vi "ConfigDevice.vi"(8 "error in (no error)":errorcluster, 11 "ChromaPowerSupply in":refnum<class "ChromaPowerSupply.lvclass">) -> (0 "error out":errorcluster, 3 "ChromaPowerSupply out":refnum<class "ChromaPowerSupply.lvclass">)   [LabVIEW 2018, in "AcPwrPlugins.lvlib" / "ChromaPowerSupply.lvclass"]
doc: "This VI configures all the properties set by the user through the INI file or the Properties Dialog box."
uses:
  ChromaPowerSupply.lvclass
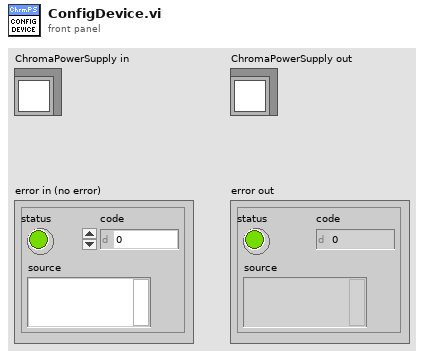
[diagram p1: front panel]
types:
  T1 = typedef "AcPwrPlugins.lvlib/ChromaPowerSupply.lvclass/Device(s)Settings.ctl" = cluster{"Phases":cluster{"Handle":string, "Instrument Options":string, "id query (T)":bool, "reset device (T)":bool, "Timing":cluster{"TimingOn":enum16{""}, "Hours":u32, "Minutes":u32, "Seconds":dbl, "CutoffVoltage":dbl}, "Connected":bool, "Output Mode":enum16{"Voltage (DC)", "Current (DC)"}, "Voltage":dbl, "Current":dbl, "High Voltage Limit":dbl, "High Current Limit":dbl, "Power Protect":dbl, "Current Protect":dbl, "Voltage Protect":dbl, "Low Current Limit":dbl, "Low Voltage Limit":dbl, "Current Slew Rate":dbl, "Voltage Slew Rate":dbl}[], "MeasName":string}
  T2 = cluster{"Handle":string, "Instrument Options":string, "id query (T)":bool, "reset device (T)":bool, "Timing":cluster{"TimingOn":enum16{""}, "Hours":u32, "Minutes":u32, "Seconds":dbl, "CutoffVoltage":dbl}, "Connected":bool, "Output Mode":enum16{"Voltage (DC)", "Current (DC)"}, "Voltage":dbl, "Current":dbl, "High Voltage Limit":dbl, "High Current Limit":dbl, "Power Protect":dbl, "Current Protect":dbl, "Voltage Protect":dbl, "Low Current Limit":dbl, "Low Voltage Limit":dbl, "Current Slew Rate":dbl, "Voltage Slew Rate":dbl}[]
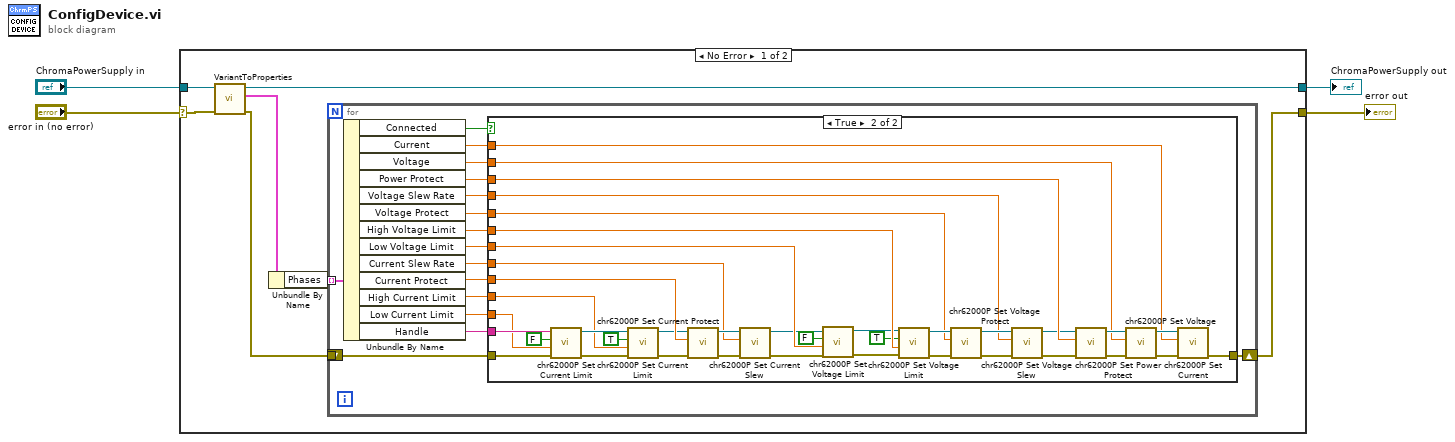
[diagram p0: block diagram]
diagram:
  n1 = case shown="No Error" "error in (no error)" {
    selector: "error in (no error)" -> [w10 w67]
    tunnel: "ChromaPowerSupply in" -> [w11 w68]
    tunnel: [w9 w68] -> w2
    tunnel: [w5 w67] -> w1
    frame No Error {
      n2 = call-dynamic "VariantToProperties.vi"("error in (no error)"=w10, "ChromaPowerSupply in"=w11) -> ("error out"=w6:errorcluster, "Device Settings"=w8:T1, "ChromaPowerSupply out"=w9:refnum<class "ChromaPowerSupply.lvclass">)  [unwired: 5 in, 2 out]
      n3 = Unbundle By Name(w8) -> ("Phases"=w7:T2)
      n4 = for {
        tunnel: w7 -> [w27] mode=indexing
        tunnel: w6 -> [w25]
        shift-right: [w22] -> w5
        shift-left: _ -> [_]
        n5 = Unbundle By Name(w27) -> ("Connected"=w18:bool, "Current"=w16:dbl, "Voltage"=w17:dbl, "Power Protect"=w19:dbl, "Voltage Slew Rate"=w12:dbl, "Voltage Protect"=w21:dbl, "High Voltage Limit"=w23:dbl, "Low Voltage Limit"=w14:dbl, "Current Slew Rate"=w13:dbl, "Current Protect"=w20:dbl, "High Current Limit"=w15:dbl, "Low Current Limit"=w24:dbl, "Handle"=w26:string)
        n6 = case shown="True" w18 {
          tunnel: w26 -> [_ w66]
          tunnel: w25 -> [w28 w65]
          tunnel: w24 -> [_ w61]
          tunnel: w23 -> [_ w64]
          tunnel: [w28 w51] -> w22
          tunnel: w21 -> [_ w57]
          tunnel: w20 -> [_ w60]
          tunnel: w19 -> [_ w56]
          tunnel: w17 -> [_ w50]
          tunnel: w16 -> [_ w49]
          tunnel: w15 -> [_ w43]
          tunnel: w14 -> [_ w40]
          tunnel: w13 -> [_ w36]
          tunnel: w12 -> [_ w29]
          frame False {
          }
          frame True {
            n7 = call <instrlib>:"chr62000P Set Current Limit.vi"("error in (no error)"=w65, "Current Limit (0.0)"=w61, "High/Low (Low)"=FALSE, "instrument handle"=w66) -> ("error out"=w48:errorcluster, "instrument handle out"=w47:refnum<k15>)  [unwired: 6 in]
            n8 = call <instrlib>:"chr62000P Set Current Limit.vi"("error in (no error)"=w48, "Current Limit (0.0)"=w43, "High/Low (Low)"=TRUE, "instrument handle"=w47) -> ("error out"=w45:errorcluster, "instrument handle out"=w46:refnum<k15>)  [unwired: 6 in]
            n9 = call <instrlib>:"chr62000P Set Current Protect.vi"("error in (no error)"=w45, "Current Protect (63.0)"=w60, "instrument handle"=w46) -> ("error out"=w38:errorcluster, "instrument handle out"=w37:refnum<k15>)  [unwired: 7 in]
            n10 = call <instrlib>:"chr62000P Set Current Slew.vi"("error in (no error)"=w38, "Current Slew (1.00)"=w36, "instrument handle"=w37) -> ("error out"=w34:errorcluster, "instrument handle out"=w35:refnum<k15>)  [unwired: 7 in]
            n11 = call <instrlib>:"chr62000P Set Voltage Limit.vi"("error in (no error)"=w34, "Voltage Limit (0.0)"=w40, "High/Low (Low)"=FALSE, "instrument handle"=w35) -> ("error out"=w41:errorcluster, "instrument handle out"=w42:refnum<k15>)  [unwired: 6 in]
            n12 = call <instrlib>:"chr62000P Set Voltage Limit.vi"("error in (no error)"=w41, "Voltage Limit (0.0)"=w64, "High/Low (Low)"=TRUE, "instrument handle"=w42) -> ("error out"=w59:errorcluster, "instrument handle out"=w58:refnum<k15>)  [unwired: 6 in]
            n13 = call <instrlib>:"chr62000P Set Voltage Protect.vi"("error in (no error)"=w59, "Voltage Protect (88.0)"=w57, "instrument handle"=w58) -> ("error out"=w33:errorcluster, "instrument handle out"=w32:refnum<k15>)  [unwired: 7 in]
            n14 = call <instrlib>:"chr62000P Set Voltage Slew.vi"("error in (no error)"=w33, "Voltage Slew (1.00)"=w29, "instrument handle"=w32) -> ("error out"=w31:errorcluster, "instrument handle out"=w30:refnum<k15>)  [unwired: 7 in]
            n15 = call <instrlib>:"chr62000P Set Power Protect.vi"("error in (no error)"=w31, "Power Protect (1260.0)"=w56, "instrument handle"=w30) -> ("error out"=w54:errorcluster, "instrument handle out"=w55:refnum<k15>)  [unwired: 7 in]
            n16 = call <instrlib>:"chr62000P Set Voltage.vi"("error in (no error)"=w54, "Voltage (0.00)"=w50, "instrument handle"=w55) -> ("error out"=w52:errorcluster, "instrument handle out"=w53:refnum<k15>)  [unwired: 7 in]
            n17 = call <instrlib>:"chr62000P Set Current.vi"("error in (no error)"=w52, "Current (0.00)"=w49, "instrument handle"=w53) -> ("error out"=w51:errorcluster)  [unwired: 7 in, 1 out]
          }
        }
      }
    }
    frame Error {
    }
  }
  "error out" <- w1
  "ChromaPowerSupply out" <- w2
